vi "Project Parser_Identify External Dependencies.vi"(7 "To Lower Case?(T)":bool=TRUE, 10 "External Folder Names":string[](array[string]), 11 "External Target Map":map{string, string}(c390)) -> (3 "Found External Dependencies":string[](array[string]))   [LabVIEW 2019, in "Project.Dependencies Finder.lvlib"]
doc: "Find folder name matches and identify the corresponding dependencies.\n\n2020-11-13: Henrik Dueholm Hansen"
uses:
  1fb010f6-fd6d-4059-9761-5e8777b5c0ce.vi
  Project.Dependencies Finder.lvlib
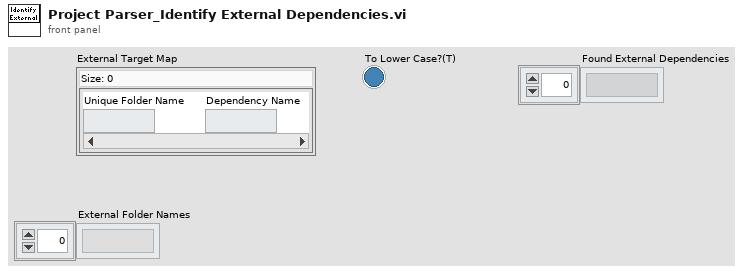
[diagram p1: front panel]
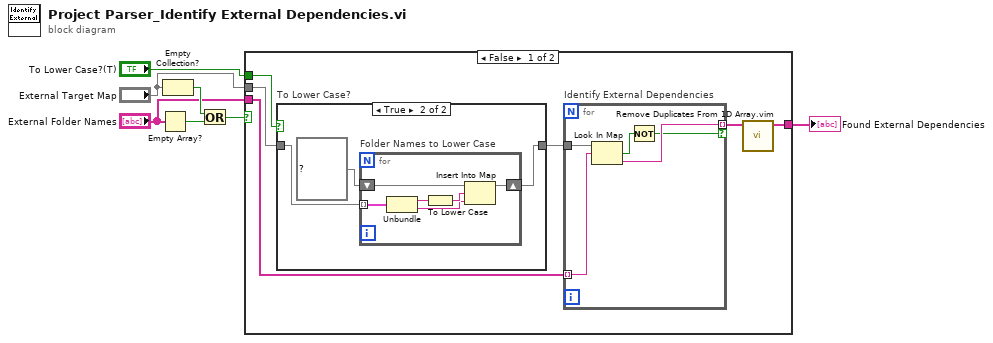
[diagram p0: block diagram]
diagram:
  n1 = Empty Array?(array="External Folder Names") -> (empty?=w2:bool)
  n2 = Empty Collection?(1:"External Target Map") -> (0:w7:bool)
  n3 = Or(x=w7, y=w2) -> (x .or. y?=w3:bool)
  n4 = case shown="False" w3 {
    tunnel: "External Target Map" -> [w13 _]
    tunnel: [w10 _] -> w5
    tunnel: "External Folder Names" -> [w9 _]
    tunnel: "To Lower Case?(T)" -> [w8 _]
    frame False {
      n5 = case "To Lower Case?" shown="True" w8 {
        tunnel: w13 -> [w14 w17]
        tunnel: [w14 w15] -> w12
        frame False {
        }
        frame True {
          n6 = for "Folder Names to Lower Case" {
            tunnel: w17 -> [w23] mode=indexing
            shift-right: [w20] -> w15
            shift-left: map{string, string} {} ("External Target Map") -> [w21]
            n7 = Unbundle(w23) -> ("Unique Folder Name"=w22:string, "Dependency Name"=w18:string)
            n8 = To Lower Case(string=w22) -> (all lower case string=w19:string)
            n9 = Insert Into Map(map in=w21, key=w19, value=w18) -> (map out=w20:map{string, string})  [unwired: 2 out]
          }
        }
      }
      n10 = for "Identify External Dependencies" {
        tunnel: w9 -> [w27] mode=indexing
        tunnel: w12 -> [w28]
        tunnel: [w25] -> w11 mode=indexing if=w24
        n11 = Look In Map(map=w28, key=w27) -> (key not found?=w26:bool, value=w25:string)  [unwired: 1 in]
        n12 = Not(x=w26) -> (.not. x?=w24:bool)
      }
      n13 = call "Remove Duplicates From 1D Array.vim"("array"=w11) -> ("array with duplicates removed"=w10:string[])  [unwired: 10 in]
    }
    frame True {
    }
  }
  "Found External Dependencies" <- w5
